vi "Teleop (3).vi"(10 "Match Info":T1={"Autonomous Elapsed Seconds"=0.0, "TeleOp Elapsed Seconds"=0.0, "Disabled Elapsed Seconds"=0.0, "Visited Autonomous"=FALSE, "Visited TeleOp"=FALSE, "Visited Disabled"=FALSE, "Autonomous Settings"={"Autonomous Style"=enum."Independent", "VI Refnum"=refnum}}, 11 "Call Context":T2) -> ()   [LabVIEW 2016]
doc: "This VI is called for each TeleOp packet received from the DS where the robot is not disabled. It is often used to read from the joysticks and update I/O or to update setpoints for timed control loops. It should complete and return within 20 milliseconds or it may miss DS packets."
uses:
  <vilib>/Rock Robotics/WPI/DriverStation/WPI_DriverStationDerivedRobotMode.ctl
  <vilib>/Rock Robotics/WPI/DriverStation/WPI_DriverStationMatch Info.ctl
  <vilib>/Rock Robotics/WPI/Solenoid/WPI_SolenoidValue.ctl
  <vilib>/Rock Robotics/WPI/Utilities/WPI_GetSetVariantRefNum.vi
  <vilib>/Rock Robotics/WPI/Joystick/WPI_JoystickArcadeMapping.vi
panel:
  out "Brake is Enabled 6":bool
  out "Brake is Enabled 5":bool
  out "Brake is Enabled 4":bool
  out "Brake is Enabled 3":bool
  out "Brake is Enabled 2":bool
  out "Brake is Enabled":bool
  out "Shift Status":dbl
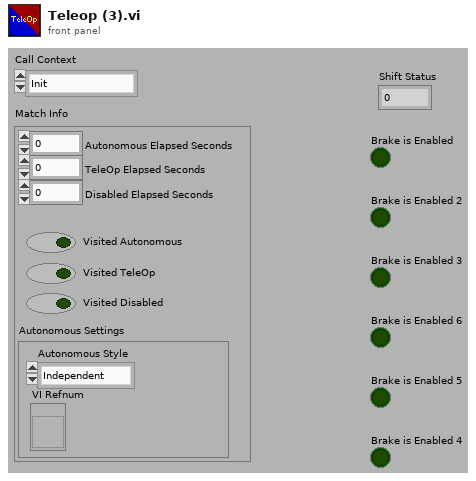
[diagram p1: front panel]
types:
  T1 = typedef "WPI_DriverStationMatch Info.ctl" = cluster{"Autonomous Elapsed Seconds":dbl, "TeleOp Elapsed Seconds":dbl, "Disabled Elapsed Seconds":dbl, "Visited Autonomous":bool, "Visited TeleOp":bool, "Visited Disabled":bool, "Autonomous Settings":cluster{"Autonomous Style":enum16{"Iterative", "Independent"}, "VI Refnum":refnum<vi>}}
  T2 = typedef "WPI_DriverStationDerivedRobotMode.ctl" = enum16{"Init", "Execute", "Stop"}
  T3 = typedef "WPI_SolenoidValue.ctl" = enum16{"Off", "On", "Forward", "Reverse"}
  T4 = typedef "WPI_JoystickDevRef.ctl" = cluster{"Device":T5}
  T5 = typedef "WPI_JoystickDeviceEnum.ctl" = enum16{"USB 0", "USB 1", "USB 2", "USB 3", "USB 4", "USB 5"}
  T6 = typedef "WPI_MotorControlDeviceRef.ctl" = cluster{"DeviceStatus":errorcluster, "Type":T7, "PWM":cluster{"PWM Channel":T8, "DeadBand":T9}, "CAN":cluster{"Device Number":u8, "SetOutput VI Ref":variant, "GetOutput VI Ref":variant, "Enable VI Ref":variant, "Disable VI Ref":variant, "Data":variant}, "Invert":bool}
  T7 = typedef "WPI_MotorControlType.ctl" = enum16{"PWM", "CAN"}
  T8 = typedef "FPGA_DIOPWMChannel.ctl" = enum8{"PWM 0", "PWM 1", "PWM 2", "PWM 3", "PWM 4", "PWM 5", "PWM 6", "PWM 7", "PWM 8", "PWM 9", "PWM MXP 0", "PWM MXP 1", "PWM MXP 2", "PWM MXP 3", "PWM MXP 4", "PWM MXP 5", "PWM MXP 6", "PWM MXP 7", "PWM MXP 8", "PWM MXP 9", "Invalid"}
  T9 = typedef "WPI_PWMDeadband.ctl" = cluster{"Name":string, "maxPositivePwm":i32, "minPositivePwm":i32, "centerPwm":i32, "maxNegativePwm":i32, "minNegativePwm":i32, "angularRange":u16}
  T10 = typedef "WPI_CANTalonSRX_GlobalStatus.ctl" = cluster{"Applied Throttle":dbl, "Module Enabled":bool, "CAN Error":errorcluster, "Closed Loop Error":dbl, "Forward Limit Switch Closed":bool, "Reverse Limit Switch Closed":bool, "Sensor Position":dbl, "Sensor Velocity":dbl, "Current":dbl, "Sticky Fault - Over Temp":bool, "Sticky Fault - Under Voltage":bool, "Sticky Fault - Forward Limit":bool, "Sticky Fault - Reverse Limit":bool, "Sticky Fault - Forward Soft Limit":bool, "Sticky Fault - Reverse Soft Limit":bool, "Brake is Enabled":bool, "Encoder Position":dbl, "Encoder Velocity":dbl, "Encoder Index Count":dbl, "Encoder A Pin State":bool, "Encoder B Pin State":bool, "Encoder Index Pin State":bool, "Analog In":dbl, "Analog In Velocity":dbl, "Temperature (C)":dbl, "Battery Voltage":dbl, "Control 5 Is Supported":bool, "Current Profile Slot Select":dbl, "Pos Div 8":bool, "Vel Div 4":bool, "Pulse Width Position":i32, "Pulse Width Velocity":i32, "Pulse Width Rise To Rise (us)":i32, "Pulse Width Rise To Fall (us)":i32, "Mot Prof Active Is Under Run":bool, "Mot Prof Active Has Under Run":bool, "Mot Prof Active Is Last":bool, "Mot Prof Active Velocity Only":bool, "Mot Prof Active Is Valid":bool, "Mot Prof Buffer Is Full":bool, "Mot Prof Active Profile Slot Select":i32, "Mot Prof NextID":i32, "Mot Prof Count":i32, "Mot Prof Active Velocity":dbl, "Mot Prof Active Position":dbl, "Mot Prof Output Enable":i32}
  T11 = typedef "WPI_SolenoidDevRef.ctl" = cluster{"DevStatus":errorcluster, "Pneumatics Control Module":u8, "Forward Solenoid Channel":T12, "Reverse Solenoid Channel":T12}
  T12 = typedef "WPI_SolenoidChannel.ctl" = enum8{"Solenoid 0", "Solenoid 1", "Solenoid 2", "Solenoid 3", "Solenoid 4", "Solenoid 5", "Solenoid 6", "Solenoid 7", "Invalid"}
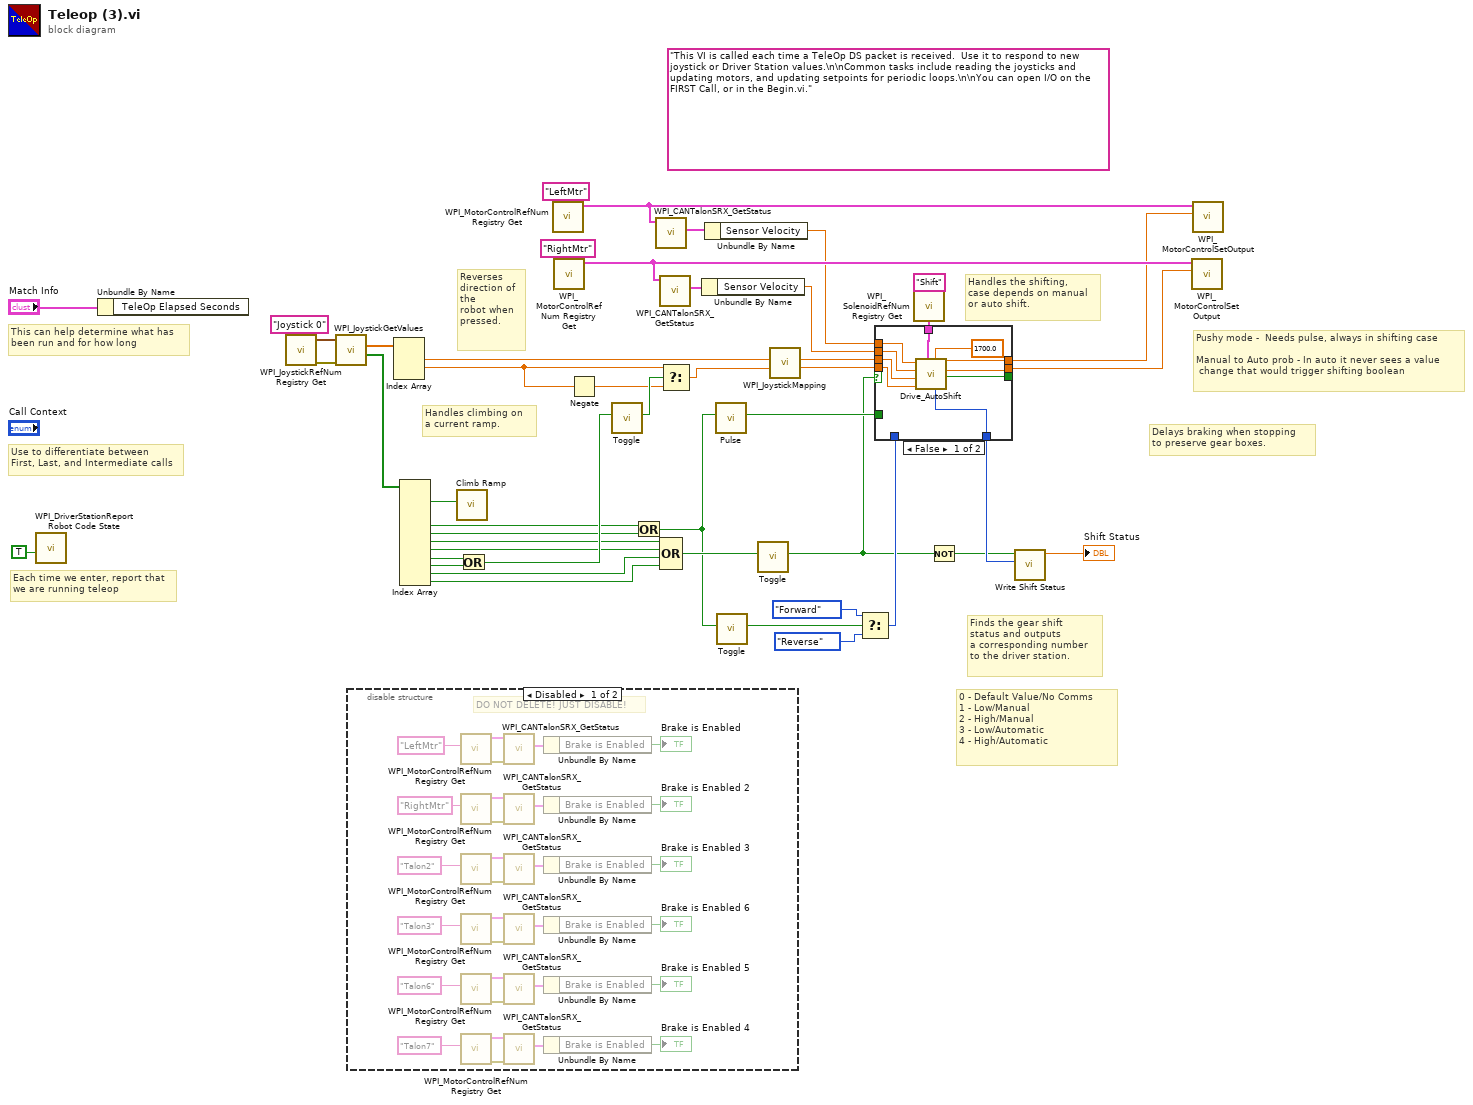
[diagram p0: block diagram]
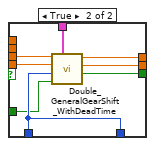
[diagram p3: hidden frame]
diagram:
  (unwired) "This VI is called each time a TeleOp DS packet is received.  Use it to respond to new joystick or Driver Station values.\n\nCommon tasks include reading the joysticks and updating motors, and updating setpoints for periodic loops.\n\nYou can open I/O on the FIRST Call, or in the Begin.vi."
  # "Pushy mode -  Needs pulse, always in shifting case\n\nManual to Auto prob - In auto it never sees a value\n change that would trigger shifting boolean"
  # "Handles the shifting,\ncase depends on manual\nor auto shift."
  # "Reverses direction of the\nrobot when pressed."
  # "Handles climbing on\na current ramp."
  # "Finds the gear shift\nstatus and outputs\na corresponding number\nto the driver station."
  # "Delays braking when stopping \nto preserve gear boxes."
  # "0 - Default Value/No Comms\n1 - Low/Manual\n2 - High/Manual\n3 - Low/Automatic\n4 - High/Automatic"
  # "Each time we enter, report that\nwe are running teleop"
  # "Use to differentiate between\nFirst, Last, and Intermediate calls"
  # "This can help determine what has\nbeen run and for how long"
  n1 = call <vilib>:"WPI_DriverStationReport Robot Code State.vi"("TeleOp"=TRUE ("Autonomous")) -> ()  [unwired: 10 in, 1 out]
  n2 = Unbundle By Name("Match Info") -> ()  [unwired: 1 out]
  n3 = call <vilib>:"WPI_JoystickRefNum Registry Get.vi"("refnum name"="Joystick 0") -> ("error out"=w41:errorcluster, "JoystickDevRef"=w45:T4)  [unwired: 1 in, 8 out]
  n4 = call <vilib>:"WPI_JoystickGetValues.vi"("error in (no error)"=w41, "JoystickDevRef"=w45) -> ("Buttons"=w42:bool[], "Axes"=w43:dbl[])  [unwired: 5 in, 3 out]
  n5 = disable-structure shown="Disabled" {
    frame Disabled {
      # "DO NOT DELETE! JUST DISABLE!"
      n6 = call <vilib>:"WPI_MotorControlRefNum Registry Get.vi"("refnum name"="LeftMtr") -> ("error out"=w69:errorcluster, "MotorControlDevRef"=w70:T6)  [unwired: 9 in]
      n7 = call <vilib>:"WPI_MotorControlRefNum Registry Get.vi"("refnum name"="RightMtr") -> ("error out"=w55:errorcluster, "MotorControlDevRef"=w54:T6)  [unwired: 9 in]
      n8 = call <vilib>:"WPI_MotorControlRefNum Registry Get.vi"("refnum name"="Talon2") -> ("error out"=w57:errorcluster, "MotorControlDevRef"=w56:T6)  [unwired: 9 in]
      n9 = call <vilib>:"WPI_MotorControlRefNum Registry Get.vi"("refnum name"="Talon3") -> ("error out"=w53:errorcluster, "MotorControlDevRef"=w52:T6)  [unwired: 9 in]
      n10 = call <vilib>:"WPI_MotorControlRefNum Registry Get.vi"("refnum name"="Talon6") -> ("error out"=w50:errorcluster, "MotorControlDevRef"=w51:T6)  [unwired: 9 in]
      n11 = call <vilib>:"WPI_MotorControlRefNum Registry Get.vi"("refnum name"="Talon7") -> ("error out"=w48:errorcluster, "MotorControlDevRef"=w49:T6)  [unwired: 9 in]
      n12 = call <vilib>:"WPI_CANTalonSRX_GetStatus.vi"("error in (no error)"=w69, "CAN Talon SRX Ref"=w70) -> ("Talon SRX Status"=w71:T10)  [unwired: 7 in, 2 out]
      n13 = call <vilib>:"WPI_CANTalonSRX_GetStatus.vi"("error in (no error)"=w55, "CAN Talon SRX Ref"=w54) -> ("Talon SRX Status"=w66:T10)  [unwired: 7 in, 2 out]
      n14 = call <vilib>:"WPI_CANTalonSRX_GetStatus.vi"("error in (no error)"=w57, "CAN Talon SRX Ref"=w56) -> ("Talon SRX Status"=w65:T10)  [unwired: 7 in, 2 out]
      n15 = call <vilib>:"WPI_CANTalonSRX_GetStatus.vi"("error in (no error)"=w53, "CAN Talon SRX Ref"=w52) -> ("Talon SRX Status"=w58:T10)  [unwired: 7 in, 2 out]
      n16 = call <vilib>:"WPI_CANTalonSRX_GetStatus.vi"("error in (no error)"=w50, "CAN Talon SRX Ref"=w51) -> ("Talon SRX Status"=w61:T10)  [unwired: 7 in, 2 out]
      n17 = call <vilib>:"WPI_CANTalonSRX_GetStatus.vi"("error in (no error)"=w48, "CAN Talon SRX Ref"=w49) -> ("Talon SRX Status"=w62:T10)  [unwired: 7 in, 2 out]
      n18 = Unbundle By Name(w71) -> ("Brake is Enabled"=→"Brake is Enabled":bool)
      n19 = Unbundle By Name(w66) -> ("Brake is Enabled"=→"Brake is Enabled 2":bool)
      n20 = Unbundle By Name(w65) -> ("Brake is Enabled"=→"Brake is Enabled 3":bool)
      n21 = Unbundle By Name(w58) -> ("Brake is Enabled"=→"Brake is Enabled 6":bool)
      n22 = Unbundle By Name(w61) -> ("Brake is Enabled"=→"Brake is Enabled 5":bool)
      n23 = Unbundle By Name(w62) -> ("Brake is Enabled"=→"Brake is Enabled 4":bool)
    }
    frame Enabled {
    }
  }
  n24 = Index Array(array=w43) -> (element #1=w27:dbl, element #2=w29:dbl)  [unwired: 3 in, 1 out]
  n25 = Index Array(array=w42) -> (element #1=w11:bool, element #4=w20:bool, element #5=w19:bool, element #6=w23:bool, element #7=w24:bool, element #8=w39:bool, element #9=w40:bool, element #10=w22:bool, element #11=w21:bool)  [unwired: 11 in, 2 out]
  n26 = call "Climb Ramp.vi"("Climb"=w11) -> ()  [unwired: 11 in]
  n27 = Or(x=w39, y=w40) -> (x .or. y?=w38:bool)
  n28 = call <vilib>:"WPI_MotorControlRefNum Registry Get.vi"("refnum name"="LeftMtr") -> ("MotorControlDevRef"=w17:T6)  [unwired: 9 in, 1 out]
  n29 = call <vilib>:"WPI_MotorControlRefNum Registry Get.vi"("refnum name"="RightMtr") -> ("MotorControlDevRef"=w16:T6)  [unwired: 9 in, 1 out]
  n30 = Negate(x=w29) -> (-x=w25:dbl)
  n31 = call "Toggle.vi"("Input"=w38) -> ("Output"=w28:bool)  [unwired: 10 in]
  n32 = Or(x=w20, y=w19) -> (x .or. y?=w4:bool)
  n33 = call <vilib>:"WPI_CANTalonSRX_GetStatus.vi"("CAN Talon SRX Ref"=w17) -> ("Talon SRX Status"=w15:T10)  [unwired: 8 in, 2 out]
  n34 = call <vilib>:"WPI_CANTalonSRX_GetStatus.vi"("CAN Talon SRX Ref"=w16) -> ("Talon SRX Status"=w14:T10)  [unwired: 8 in, 2 out]
  n35 = Compound Arithmetic op=OR(w23, w24, w22, w21) -> (w5:bool)
  n36 = Select(t=w29, s=w28, f=w25) -> (s? t:f=w26:dbl)
  n37 = Unbundle By Name(w14) -> ("Sensor Velocity"=w13:dbl)
  n38 = Unbundle By Name(w15) -> ("Sensor Velocity"=w8:dbl)
  n39 = call "Pulse.vi"("Input"=w4) -> ("Output"=w3:bool)  [unwired: 10 in]
  n40 = call "Toggle.vi"("Input"=w4) -> ("Output"=w33:bool)  [unwired: 10 in]
  n41 = call "Toggle.vi"("Input"=w5) -> ("Output"=w2:bool)  [unwired: 10 in]
  n42 = call-poly <vilib>:"WPI_JoystickMapping.vi"("Y axis value"=w26, "X axis value"=w27) -> ("Right Motor Value"=w31:dbl, "Left Motor Value"=w32:dbl)  [unwired: 8 in]
  n43 = Select(t=WPI_SolenoidValue."Forward" ("Value"), s=w33, f=WPI_SolenoidValue."Reverse" ("Value")) -> (s? t:f=w6:T3)
  n44 = call <vilib>:"WPI_SolenoidRefNum Registry Get.vi"("refnum name"="Shift") -> ("SolenoidDevRef"=w18:T11)  [unwired: 9 in, 1 out]
  n45 = case shown="False" w2 {
    tunnel: [w85 w95] -> w9
    tunnel: [w86 w94] -> w12
    tunnel: w32 -> [w84 w93]
    tunnel: w31 -> [w83 w92]
    tunnel: w18 -> [w79 w90]
    tunnel: [w87 w91] -> _
    tunnel: w13 -> [w82 _]
    tunnel: w8 -> [w81 _]
    tunnel: [w78 w89] -> w7
    tunnel: w6 -> [_ w89]
    tunnel: w3 -> [_ w88]
    frame False {
      n46 = call "Drive_AutoShift.vi"("Max"=1700.0, "ShifterRef"=w79, "Right  Input"=w83, "Left Input"=w84, "Right RPM"=w82, "Left RPM"=w81) -> ("Shifting"=w87:bool, "Right Output"=w86:dbl, "Left Output"=w85:dbl, "Gear"=w78:T3)  [unwired: 2 in]
    }
    frame True {
      n47 = call "Double_GeneralGearShift_WithDeadTime.vi"("ShifterRef"=w90, "Shift Control"=w88, "Shift Value"=w89, "Right"=w92, "Left"=w93) -> ("Shifting"=w91:bool, "Right Output"=w94:dbl, "Left Output"=w95:dbl)  [unwired: 3 in, 1 out]
    }
  }
  n48 = Not(x=w2) -> (.not. x?=w1:bool)
  n49 = call "Write Shift Status.vi"("Gear"=w7, "Output"=w1) -> ("Shift Status"=→"Shift Status":dbl)  [unwired: 9 in]
  n50 = call <vilib>:"WPI_MotorControlSetOutput.vi"("Output"=w12, "MotorControlDevRef"=w16) -> ()  [unwired: 7 in, 3 out]
  n51 = call <vilib>:"WPI_MotorControlSetOutput.vi"("Output"=w9, "MotorControlDevRef"=w17) -> ()  [unwired: 7 in, 3 out]
